vi "Edit Substeps Digital Input.vi"(8 "error in":errorcluster, 10 "DI In":T1, 11 "Sequence Context In":refnum<k7>) -> (0 "error out":errorcluster, 2 "DI Out":T1, 3 "Report Text":string)   [LabVIEW 2023, in "LTT_TeststandSteptypes.lvlib"]
doc: "This VI Analog Input Signal Map and Multinumberic Edit Sub step"
uses:
  LTT_TeststandSteptypes.lvlib
  HardwareAbstractionLayer_LVOOP/Digital Input/DI_class/DI DAQ/Control/DI Step Control.ctl
  HardwareAbstractionLayer_LVOOP/Database/SQL Public VI/Control/DB Options.ctl
  <vilib>/addons/TestStand/_TSUtility.llb/TestStand - Start Modal Dialog (Sequence Context).vi
  <vilib>/addons/TestStand/_TSUtility.llb/TestStand - End Modal Dialog (Sequence Context).vi
  HardwareAbstractionLayer_LVOOP/Database/Database.lvclass
  HardwareAbstractionLayer_LVOOP/Digital Input/DI_class/DI.lvclass
panel:
  in  "Close":bool
  in  "OK":bool
  in  "Station No":i32
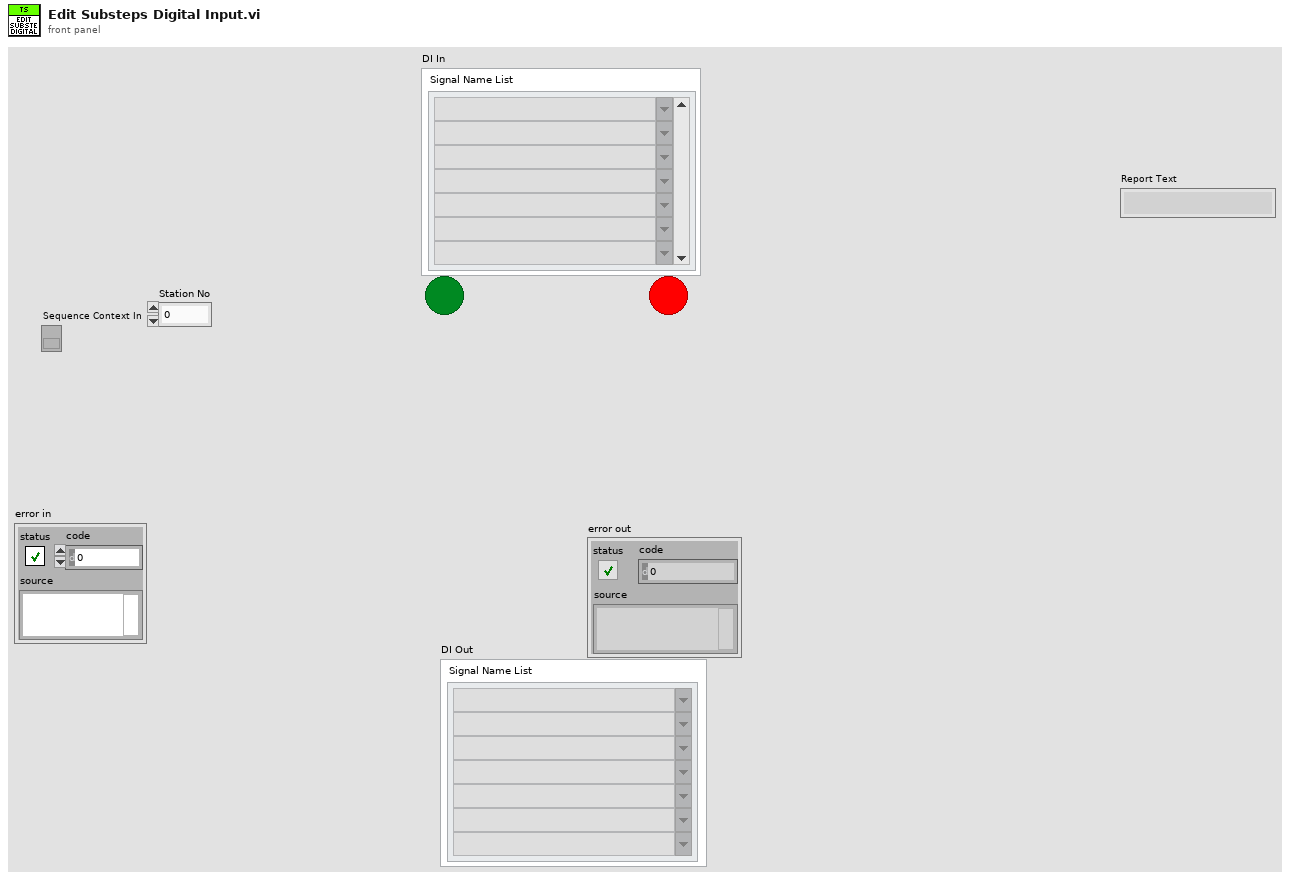
[diagram p1: front panel]
types:
  T1 = typedef "HardwareAbstractionLayer_LVOOP.lvlib/DI.lvclass/DI Step Control.ctl" = cluster{"Signal Name List":string[]}
  T2 = typedef "HardwareAbstractionLayer_LVOOP.lvlib/Database.lvclass/DB Options.ctl" = enum16{"Init", "Select Data", "Insert Data", "Update Data", "Delete Data", "Execute Query", "Create Schema", "Create Table", "List Tables", "List Columns", "Close"}
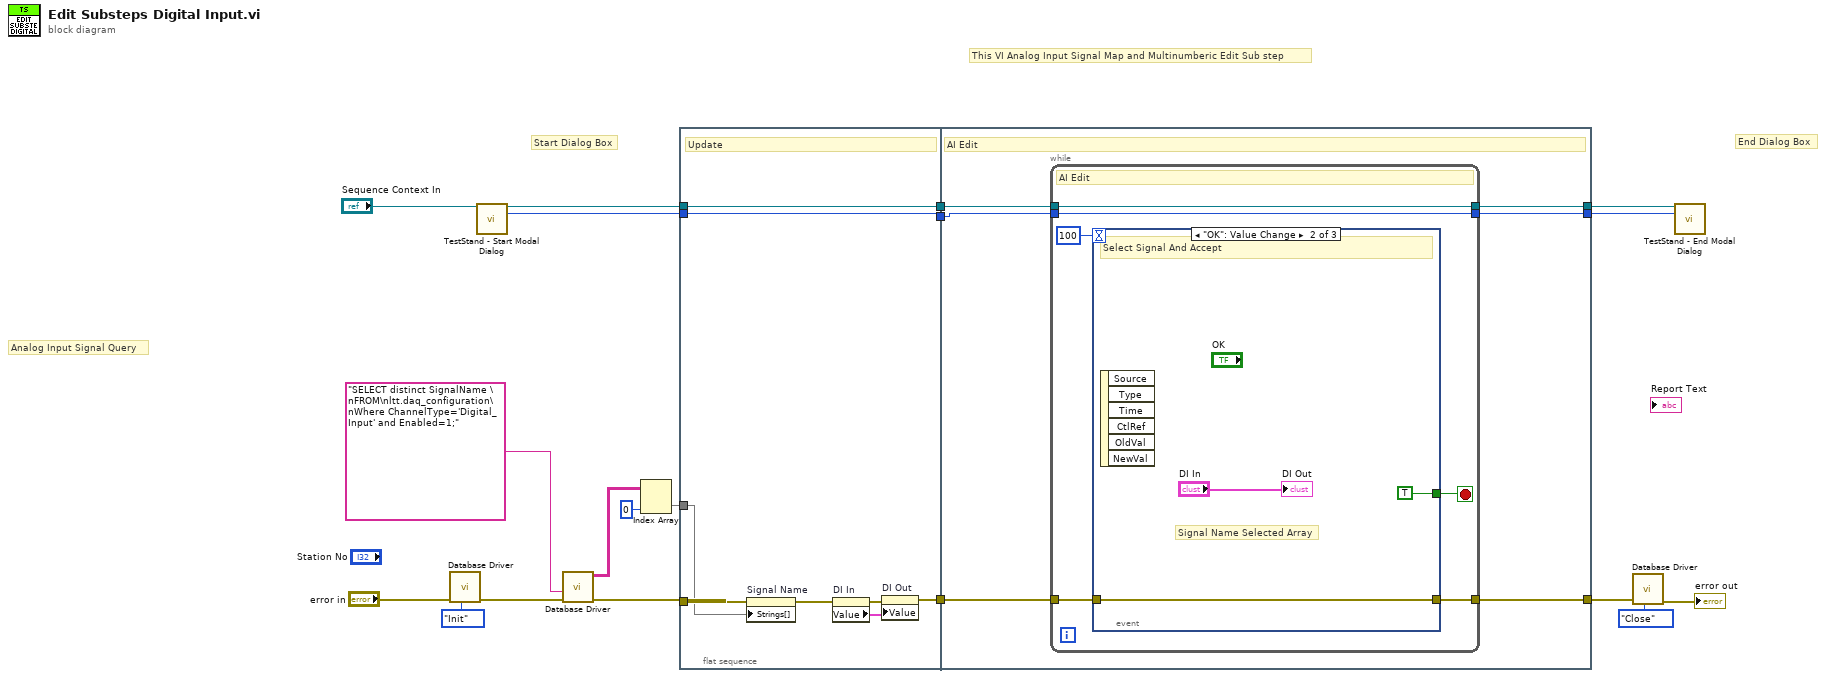
[diagram p0: block diagram]
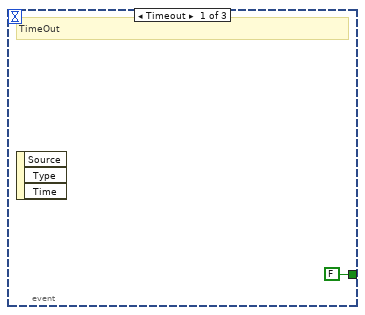
[diagram p2: hidden frame]
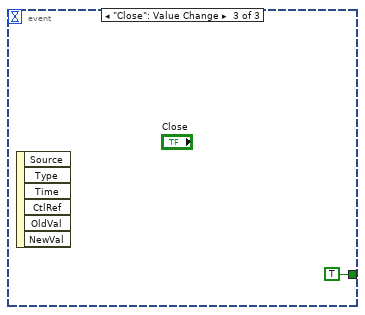
[diagram p3: hidden frame]
diagram:
  # "Analog Input Signal Query"
  # "This VI Analog Input Signal Map and Multinumberic Edit Sub step"
  # "End Dialog Box"
  # "Start Dialog Box"
  n1 = call "Database Driver.vi"("Options"=DB_Options."Init", "error in"="error in") -> ("error out"=w7:errorcluster)  [unwired: 6 in, 3 out]
  n2 = call-poly <vilib>:"TestStand - Start Modal Dialog.vi"("Sequence Context In"="Sequence Context In") -> ("Sequence Context Out"=w18:refnum<k7>, "Modal ID"=w17:i32)  [unwired: 10 in, 3 out]
  n3 = call "Database Driver.vi"("error in"=w7, "SQL query"="SELECT distinct SignalName \nFROM\nltt.daq_configuration\nWhere ChannelType='Digital_Input' and Enabled=1;") -> ("error out"=w9:errorcluster, "data"=w12:string[][])  [unwired: 6 in, 2 out]
  n4 = Index Array(array=w12, index (col)=0 ("disabled index (col)")) -> (element=w10:string[])  [unwired: 1 in]
  n5 = flat-sequence {
    tunnel: w9 -> [w23]
    tunnel: w10 -> [w24]
    tunnel: w18 -> [w27]
    tunnel: w17 -> [w26]
    tunnel: [w27] -> w16
    tunnel: [w26] -> w15
    tunnel: [w20] -> w2
    tunnel: w16 -> [w33]
    tunnel: [w32] -> w14
    tunnel: w15 -> [w31]
    tunnel: [w30] -> w13
    tunnel: w2 -> [w29]
    tunnel: [w28] -> w1
    frame #0 {
      # "Update"
      n6 = property on="Signal Name" class="CmbBox"(error in=w23, "Strings[]"=w24) -> (error out=w22:errorcluster)  [unwired: 1 in, 1 out]
      n7 = property on="DI In" class="Clust (strict)"(error in=w22) -> (error out=w21:errorcluster, "Value"=w25:T1)  [unwired: 1 in, 1 out]
      n8 = property on="DI Out" class="Clust (strict)"(error in=w21, "Value"=w25) -> (error out=w20:errorcluster)  [unwired: 1 in, 1 out]
    }
    frame #1 {
      # "AI Edit"
      n9 = while {
        tunnel: w33 -> [w39]
        tunnel: [w39] -> w32
        tunnel: w31 -> [w38]
        tunnel: [w38] -> w30
        tunnel: w29 -> [w35]
        tunnel: [w34] -> w28
        stop <- w36 stop-if-true
        # "AI Edit"
        n10 = event shown="[1] \"OK\": Value Change" {
          selector: _ -> [_ _ _]
          dyn-events: _ -> [_ _ _]
          timeout: 100 -> [_ _ _]
          tunnel: [FALSE TRUE TRUE] -> w36
          tunnel: w35 -> [_ w41 _]
          tunnel: [_ w41 _] -> w34
          event Timeout {
            # "TimeOut"
            n11 = event-data() -> ()  [unwired: 1 in, 3 out]
          }
          event "OK": Value Change {
            # "Signal Name Selected Array"
            # "Select Signal And Accept"
            n12 = event-data() -> ()  [unwired: 1 in, 6 out]
            "DI Out" <- "DI In"
          }
          event "Close": Value Change {
            n13 = event-data() -> ()  [unwired: 1 in, 6 out]
          }
        }
      }
    }
  }
  n14 = call "Database Driver.vi"("Options"=DB_Options."Close", "error in"=w1) -> ("error out"=→"error out":errorcluster)  [unwired: 6 in, 3 out]
  n15 = call-poly <vilib>:"TestStand - End Modal Dialog.vi"("Sequence Context In"=w14, "Modal ID"=w13) -> ()  [unwired: 13 in, 1 out]
